vi "GetSlotNr.vi"(8 "Error In":errorcluster, 10 "Variable In":string, 11 "Variant In":variant) -> (0 "Error Out":errorcluster, 2 "Nr of Slots Out":i32, 3 "Variant Out":variant)   [LabVIEW 2011]
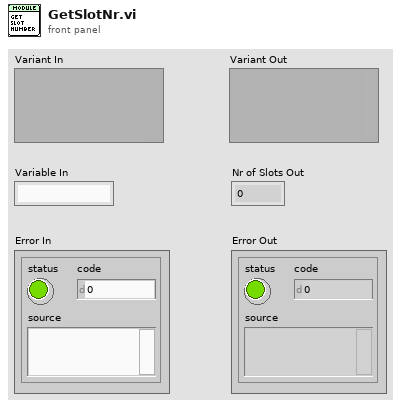
[diagram p1: front panel]
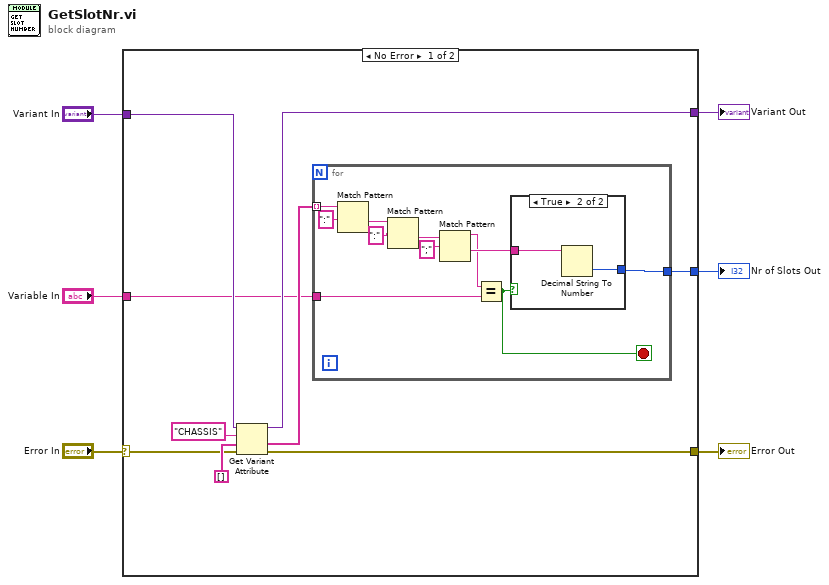
[diagram p0: block diagram]
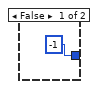
[diagram p2: hidden frame]
diagram:
  n1 = case shown="No Error" "Error In" {
    selector: "Error In" -> [w7 w30]
    tunnel: "Variant In" -> [w13 _]
    tunnel: [w12 _] -> w5
    tunnel: "Variable In" -> [w10 _]
    tunnel: [w9 _] -> w3
    tunnel: [w8 w30] -> w2
    frame No Error {
      n2 = Get Variant Attribute(Variant=w13, name="CHASSIS", default value (empty Variant)=string[] [], error in=w7) -> (duplicate Variant=w12:variant, value=w11:string[], error out=w8:errorcluster)  [unwired: 1 out]
      n3 = for {
        tunnel: w11 -> [w17] mode=indexing
        tunnel: w10 -> [w25]
        tunnel: [w24] -> w9
        stop <- w23 stop-if-true
        n4 = Match Pattern(string=w17, regular expression=":") -> (after substring=w16:string)  [unwired: 1 in, 3 out]
        n5 = Match Pattern(string=w16, regular expression=":") -> (after substring=w21:string)  [unwired: 1 in, 3 out]
        n6 = Match Pattern(string=w21, regular expression=";") -> (before substring=w19:string, after substring=w20:string)  [unwired: 1 in, 2 out]
        n7 = Equal?(x=w19, y=w25) -> (x = y?=w23:bool)
        n8 = case shown="True" w23 {
          tunnel: w20 -> [_ w28]
          tunnel: [-1 w29] -> w24
          frame False {
          }
          frame True {
            n9 = Decimal String To Number(string=w28) -> (number=w29:i32)  [unwired: 2 in, 1 out]
          }
        }
      }
    }
    frame Error {
    }
  }
  "Variant Out" <- w5
  "Nr of Slots Out" <- w3
  "Error Out" <- w2
